vi "Data read.vi"(7 "Timeout [ms]":dbl=5000.0, 8 "error in (no error)":errorcluster, 9 "Data With Stability Sign":bool, 10 "Decode Status (F)/ Decode Data (T)":bool, 11 "VISA resource name":refnum<visa-resource-name>) -> (0 "error out":errorcluster, 1 "Unit":string, 2 "Value":dbl, 3 "VISA resource name out":refnum<visa-resource-name>, 4 "Stability Sign":string="-", 5 "ID":string, 6 "Status":string)   [LabVIEW 2017, in "RadWag balances and scales.lvlib"]
doc: "Gets data from serial port and decodes them in order to return requested values."
uses:
  <instrlib>/Radwag Balances and Scales/Public/RadWag balances and scales.lvlib
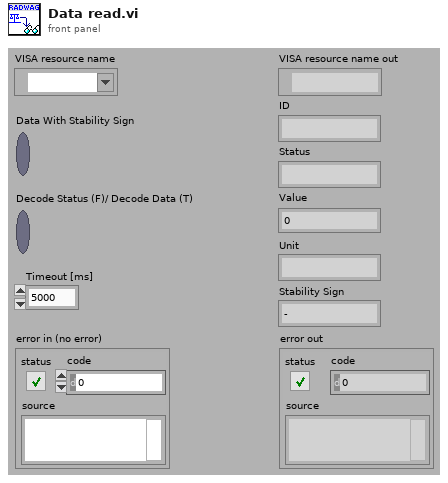
[diagram p1: front panel]
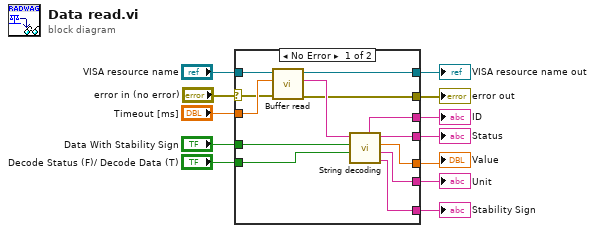
[diagram p0: block diagram]
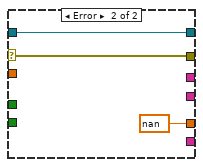
[diagram p2: hidden frame]
diagram:
  n1 = case shown="No Error" "error in (no error)" {
    selector: "error in (no error)" -> [w17 w27]
    tunnel: "Timeout [ms]" -> [w25 _]
    tunnel: "VISA resource name" -> [w24 w28]
    tunnel: "Data With Stability Sign" -> [w23 _]
    tunnel: "Decode Status (F)/ Decode Data (T)" -> [w22 _]
    tunnel: [w20 w28] -> w7
    tunnel: [w16 _] -> w6
    tunnel: [w15 _] -> w5
    tunnel: [w19 nan ("Value")] -> w4
    tunnel: [w14 _] -> w3
    tunnel: [w13 _] -> w2
    tunnel: [w18 w27] -> w1
    frame No Error {
      n2 = call <instrlib>:"Buffer read.vi"("error in (no error)"=w17, "Timeout [ms]"=w25, "VISA resource name"=w24) -> ("error out"=w18:errorcluster, "Received String"=w21:string, "VISA resource name out"=w20:refnum<visa-resource-name>)  [unwired: 6 in]
      n3 = call <instrlib>:"String decoding.vi"("Decode Status (F)/ Decode Data (T)"=w22, "Decode Stability Sign"=w23, "Input string"=w21) -> ("Stability sign"=w14:string, "Unit"=w13:string, "Value"=w19:dbl, "Status"=w15:string, "ID"=w16:string)  [unwired: 4 in]
    }
    frame Error {
    }
  }
  "error out" <- w1
  "VISA resource name out" <- w7
  "Status" <- w5
  "Value" <- w4
  "Unit" <- w2
  "Stability Sign" <- w3
  "ID" <- w6
